vi "LoadPodMiscData.vi"(9 "Pod Number":i32, 10 "Pod Configuration in":T2, 11 "Config File Refnum in":T1) -> (2 "Pod Configuration out":T2, 3 "Config File Refnum out":T1)   [LabVIEW 2014]
uses:
  <vilib>/Utility/config.llb/Config Data RefNum.ctl
  <vilib>/Utility/config.llb/Read Key (I32).vi
  <vilib>/Utility/config.llb/Write Key (I32).vi
  <vilib>/Utility/config.llb/Read Key (Double).vi
  <vilib>/Utility/config.llb/Write Key (Double).vi
  <vilib>/Utility/config.llb/NI_LVConfig.lvlib
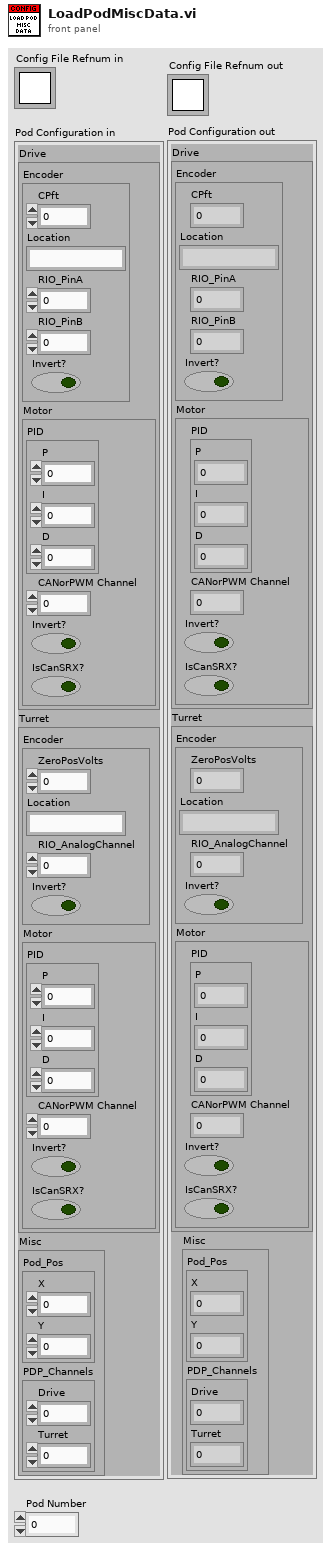
[diagram p1: front panel]
types:
  T1 = typedef "NI_LVConfig.lvlib/Config Data RefNum.ctl" = refnum<k1>
  T2 = cluster{"Drive":cluster{"Encoder":cluster{"CPft":dbl, "Location":string, "RIO_PinA":i32, "RIO_PinB":i32, "Invert?":bool}, "Motor":cluster{"PID":cluster{"P":dbl, "I":dbl, "D":dbl}, "CANorPWM Channel":i32, "Invert?":bool, "IsCanSRX?":bool}}, "Turret":cluster{"Encoder":cluster{"ZeroPosVolts":dbl, "Location":string, "RIO_AnalogChannel":i32, "Invert?":bool}, "Motor":cluster{"PID":cluster{"P":dbl, "I":dbl, "D":dbl}, "CANorPWM Channel":i32, "Invert?":bool, "IsCanSRX?":bool}}, "Misc":cluster{"Pod_Pos":cluster{"X":dbl, "Y":dbl}, "PDP_Channels":cluster{"Drive":i32, "Turret":i32}}}
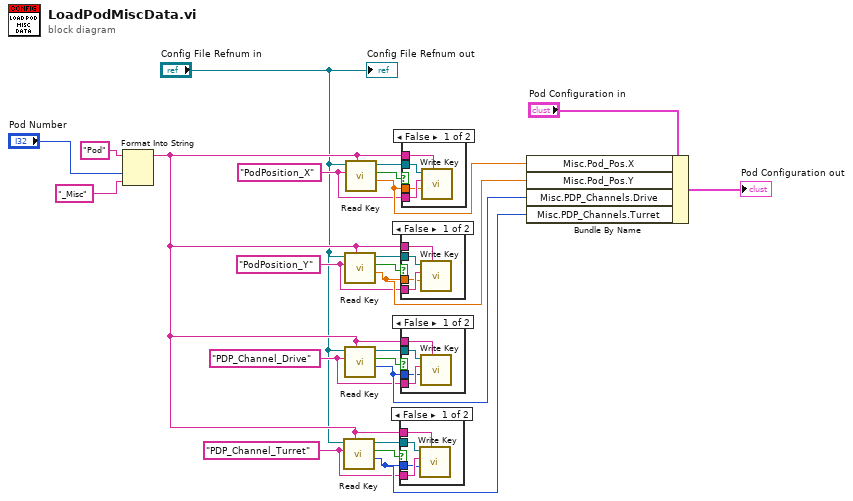
[diagram p0: block diagram]
diagram:
  w17 = "PDP_Channel_Turret" ("string")
  w20 = "PDP_Channel_Drive" ("string")
  w5 = "PodPosition_Y" ("string")
  w2 = "PodPosition_X" ("string")
  n1 = Format Into String(initial string="Pod", "Pod Number", "_Misc") -> (resulting string=w21:string)  [unwired: 2 in, 1 out]
  n2 = call-poly <vilib>:"Read Key.vi"("section"=w21, "key"=w17, "refnum"="Config File Refnum in") -> ("value"=w23:i32, "found?"=w15:bool, "refnum out"=w16:T1)  [unwired: 5 in, 1 out]
  n3 = call-poly <vilib>:"Read Key.vi"("section"=w21, "key"=w5, "refnum"="Config File Refnum in") -> ("value"=w10:dbl, "found?"=w7:bool, "refnum out"=w6:T1)  [unwired: 5 in, 1 out]
  n4 = call-poly <vilib>:"Read Key.vi"("section"=w21, "key"=w20, "refnum"="Config File Refnum in") -> ("value"=w22:i32, "found?"=w18:bool, "refnum out"=w19:T1)  [unwired: 5 in, 1 out]
  n5 = call-poly <vilib>:"Read Key.vi"("section"=w21, "key"=w2, "refnum"="Config File Refnum in") -> ("value"=w9:dbl, "found?"=w4:bool, "refnum out"=w3:T1)  [unwired: 5 in, 1 out]
  n6 = case shown="False" w15 {
    tunnel: w16 -> [w27 _]
    tunnel: w17 -> [w26 _]
    tunnel: w23 -> [w25 _]
    tunnel: w21 -> [w24 _]
    frame False {
      n7 = call-poly <vilib>:"Write Key.vi"("section"=w24, "value"=w25, "key"=w26, "refnum"=w27) -> ()  [unwired: 5 in, 3 out]
    }
    frame True {
    }
  }
  n8 = case shown="False" w7 {
    tunnel: w6 -> [w31 _]
    tunnel: w5 -> [w30 _]
    tunnel: w10 -> [w29 _]
    tunnel: w21 -> [w28 _]
    frame False {
      n9 = call-poly <vilib>:"Write Key.vi"("section"=w28, "value"=w29, "key"=w30, "refnum"=w31) -> ()  [unwired: 5 in, 3 out]
    }
    frame True {
    }
  }
  n10 = case shown="False" w18 {
    tunnel: w19 -> [w35 _]
    tunnel: w20 -> [w34 _]
    tunnel: w22 -> [w33 _]
    tunnel: w21 -> [w32 _]
    frame False {
      n11 = call-poly <vilib>:"Write Key.vi"("section"=w32, "value"=w33, "key"=w34, "refnum"=w35) -> ()  [unwired: 5 in, 3 out]
    }
    frame True {
    }
  }
  n12 = case shown="False" w4 {
    tunnel: w3 -> [w39 _]
    tunnel: w2 -> [w38 _]
    tunnel: w9 -> [w37 _]
    tunnel: w21 -> [w36 _]
    frame False {
      n13 = call-poly <vilib>:"Write Key.vi"("section"=w36, "value"=w37, "key"=w38, "refnum"=w39) -> ()  [unwired: 5 in, 3 out]
    }
    frame True {
    }
  }
  n14 = Bundle By Name(cluster="Pod Configuration in", "Misc.Pod_Pos.X"=w9, "Misc.Pod_Pos.Y"=w10, "Misc.PDP_Channels.Drive"=w22, "Misc.PDP_Channels.Turret"=w23) -> (→"Pod Configuration out":T2)
  "Config File Refnum out" <- "Config File Refnum in"
